vi "Ej2.vi"(1 "Deg C":dbl) -> (0 "Deg F":dbl)   [LabVIEW 2023]
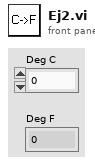
[diagram p1: front panel]
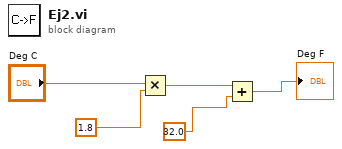
[diagram p0: block diagram]
diagram:
  n1 = Multiply(x="Deg C", y=1.8) -> (x*y=w1:dbl)
  n2 = Add(x=w1, y=32.0) -> (x+y=→"Deg F":dbl)
